vi "Black_image_detection.vi"(0 "Match score":i32[](array[numeric])) -> (1 "Black image error":bool, 2 "Image taken without error":bool)   [LabVIEW 2022 SP3]
doc: "Compares the match score from the computer vision to determine if the image were taken with or without errors."
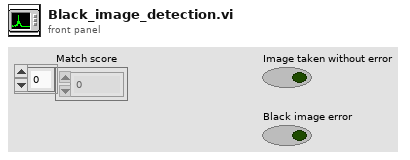
[diagram p1: front panel]
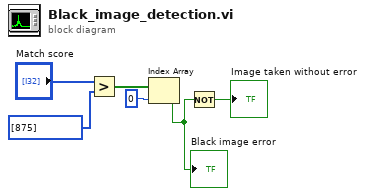
[diagram p0: block diagram]
diagram:
  n1 = Greater?(x="Match score", y=i32[] [875]) -> (0:w2:bool[])
  n2 = Index Array(array=w2, index=0) -> (element=w5:bool)
  "Black image error" <- w5
  n3 = Not(x=w5) -> (.not. x?=→"Image taken without error":bool)
